vi "niDTS GNSS GPS Rx RF Test Get Default Parameters.vi"(0 "Template Tx Test Handle in":T3, 11 "error in (no error)":errorcluster) -> (4 "Template Tx Test Handle out":T3, 8 "Default Parameters":T1 {"External Attenuation (dB)" format="%.1g"; "Power (dBm)" format="%.1g"}, 15 "error out":errorcluster)   [LabVIEW 2014, in "niDTS GNSS.lvlib"]
uses:
  niDTS GNSS.lvlib
  RF Test/Includes/niDTS GNSS RF Test INC Handle.ctl
  RF Test/Objects/BASE_class/niDTS GNSS RF Test.lvclass
  Includes/niDTS GNSS GPS Rx RF Test INC Parameters.ctl
  Includes/niDTS GNSS GPS Rx RF Test INC Channel.ctl
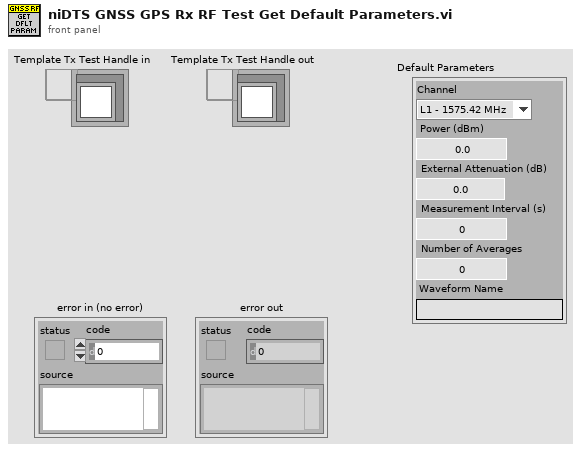
[diagram p1: front panel]
types:
  T1 = typedef "niDTS GNSS.lvlib/niDTS GNSS GPS Rx RF Test INC Parameters.ctl" = cluster{"Channel":T2, "Power (dBm)":dbl, "External Attenuation (dB)":dbl, "Measurement Interval (s)":dbl, "Number of Averages":i32, "Waveform Name":string}
  T2 = typedef "niDTS GNSS.lvlib/niDTS GNSS GPS Rx RF Test INC Channel.ctl" = enum16{"L1 - 1575.42 MHz", "L2 - 1227.60 MHz", "L5 - 1176.45 MHz"}
  T3 = typedef "niDTS GNSS.lvlib/niDTS GNSS RF Test INC Handle.ctl" = refnum<data-value>
  T4 = typedef "niDTS GNSS.lvlib/niDTS GNSS RF Test INC Parameters.ctl" = cluster{"GNSS Standard":enum16{"GPS", "GLONASS", "Galileo", "Beidou"}, "Frequency (Hz)":dbl, "Auto Level":bool, "Power (dBm)":dbl, "External Attenuation (dB)":dbl, "Measurement Interval (s)":dbl, "Pattern":enum16{"0", "1", "01", "00001111", "PN9"}, "Enable Averaging":bool, "Type Of Averaging":enum16{"MEAN", "MAX", "MIN", "MAXMIN"}, "Number of Averages":i32, "Waveform Name":string, "Enable Traces":bool}
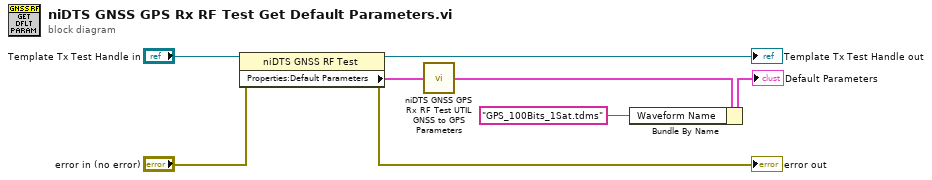
[diagram p0: block diagram]
diagram:
  n1 = property class="niDTS GNSS RF Test"(reference="Template Tx Test Handle in", error in="error in (no error)") -> (reference out=→"Template Tx Test Handle out":T3, error out=→"error out":errorcluster, "Properties:Default Parameters"=w4:T4)
  n2 = call "niDTS GNSS GPS Rx RF Test UTIL GNSS to GPS Parameters.vi"("Parameters IN"=w4) -> ("Parameters OUT"=w3:T1)
  n3 = Bundle By Name(cluster=w3, "Waveform Name"="GPS_100Bits_1Sat.tdms") -> (→"Default Parameters":T1)
